vi "filterWheelThorlabs.vi"() -> ()   [LabVIEW 2017]
panel:
  out "read buffer":string
  out "port":i32
  in  "position":u8
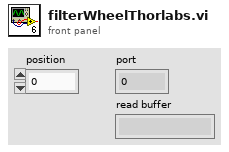
[diagram p1: front panel]
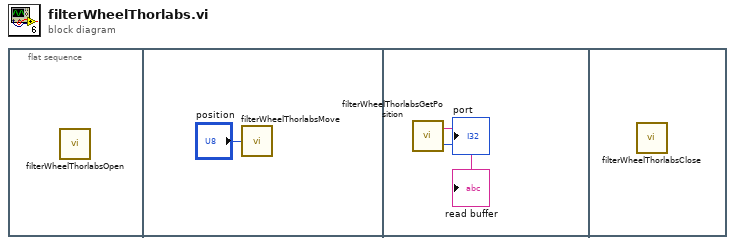
[diagram p0: block diagram]
diagram:
  n1 = flat-sequence {
    frame #0 {
      n2 = call "filterWheelThorlabsOpen.vi"() -> ()  [unwired: 12 in]
    }
    frame #1 {
      n3 = call "filterWheelThorlabsMove.vi"("position"="position") -> ()  [unwired: 1 in]
    }
    frame #2 {
      n4 = call "filterWheelThorlabsGetPosition.vi"() -> ("port"=→"port":i32, "read buffer"=→"read buffer":string)  [unwired: 2 in]
    }
    frame #3 {
      n5 = call "filterWheelThorlabsClose.vi"() -> ()  [unwired: 12 in]
    }
  }
